vi "CC FITS Filter Header Name.vi"(8 "error in (no error)":errorcluster, 11 "FITS Name In":string) -> (0 "error out":errorcluster, 3 "FITS Name Out":string)   [LabVIEW 2024]
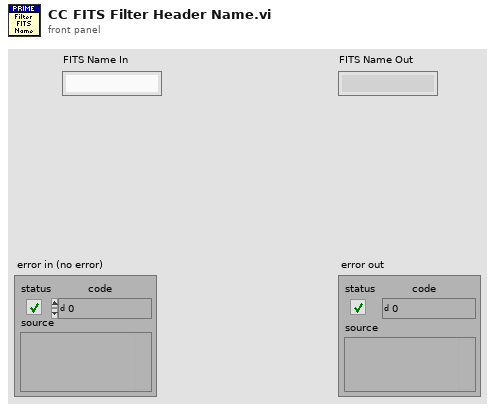
[diagram p1: front panel]
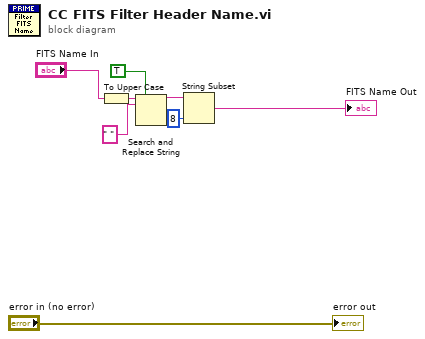
[diagram p0: block diagram]
diagram:
  n1 = To Upper Case(1:"FITS Name In") -> (0:w5:string)
  n2 = Search and Replace String(replace all?=TRUE ("replace all? (F)"), input string=w5, search string=" ") -> (result string=w4:string)  [unwired: 5 in, 3 out]
  n3 = String Subset(string=w4, length (rest)=8 ("length (rest)")) -> (substring=→"FITS Name Out":string)  [unwired: 1 in]
  "error out" <- "error in (no error)"
